vi "Prompt.vi"(11 "URL":string caption="Go to this URL then press Authorize") -> (0 "error out":errorcluster)   [LabVIEW 2010]
panel:
  in  "stop":bool
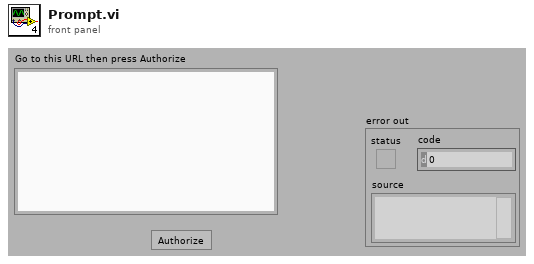
[diagram p1: front panel]
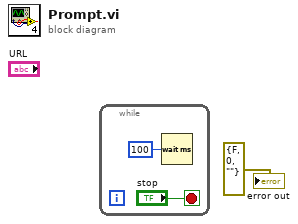
[diagram p0: block diagram]
diagram:
  n1 = while {
    stop <- "stop" stop-if-true
    n2 = Wait (ms)(milliseconds to wait=u32 100) -> ()  [unwired: 1 out]
  }
  "error out" <- errorcluster {"status"=FALSE, "code"=0, "source"=""} ("error out")
